vi "LVCAM Destroy Self.vi"(10 "Error":errorcluster, 11 "Self Actor in":refnum<class "Self Actor.lvclass">) -> (0 "error out":errorcluster, 1 "Destroyed Self?":bool, 3 "Self Actor out":refnum<class "Self Actor.lvclass">)   [LabVIEW 2021, in "LVCAM.lvlib" / "Self Actor.lvclass"]
uses:
  Self Actor.lvclass
  C:/PPLs/LabVIEW-Composed-Actor-Model-LVCAM/LabVIEW-Composed-Actor-Model-LVCAM/AAM/LVCAM/LVCAM/LVCAM.lvclass
  Self Actor.lvclass/Self Actor.ctl
  Msgs/LVCAM Destroy Self/LVCAM Destroy Self Msg/LVCAM Destroy Self Msg.lvclass
  C:/PPLs/LabVIEW-Composed-Actor-Model-LVCAM/LabVIEW-Composed-Actor-Model-LVCAM/AAM/LVCAM/Msg/Msg.lvclass
  Msgs/LVCAM Nest Destroyed/LVCAM Nest Destroyed Msg/LVCAM Nest Destroyed Msg.lvclass
  Nest Msg Send.vi
  Call Msg Send.vi
  Msg Q/Msg Q.lvclass
  C:/PPLs/LabVIEW-Composed-Actor-Model-LVCAM/LabVIEW-Composed-Actor-Model-LVCAM/AAM/Msgs/LVCAM Destroy Self/LVCAM Destroy Self Msg/LVCAM Destroy Self Msg.lvclass
  C:/PPLs/LabVIEW-Composed-Actor-Model-LVCAM/LabVIEW-Composed-Actor-Model-LVCAM/AAM/Msgs/LVCAM Destroy Self/LVCAM Destroy Self/LVCAM Destroy Self.lvclass
  C:/PPLs/LabVIEW-Composed-Actor-Model-LVCAM/LabVIEW-Composed-Actor-Model-LVCAM/AAM/Msgs/LVCAM Nest Destroyed/LVCAM Nest Destroyed Msg/LVCAM Nest Destroyed Msg.lvclass
  C:/PPLs/LabVIEW-Composed-Actor-Model-LVCAM/LabVIEW-Composed-Actor-Model-LVCAM/AAM/Msgs/LVCAM Nest Destroyed/LVCAM Nest Destroyed/LVCAM Nest Destroyed.lvclass
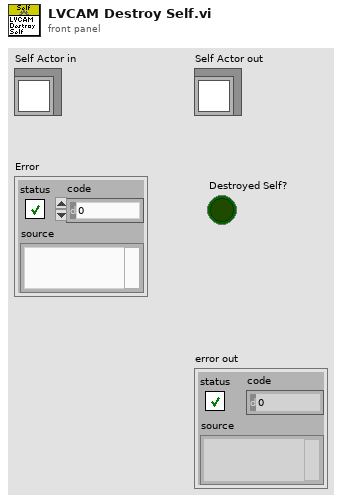
[diagram p1: front panel]
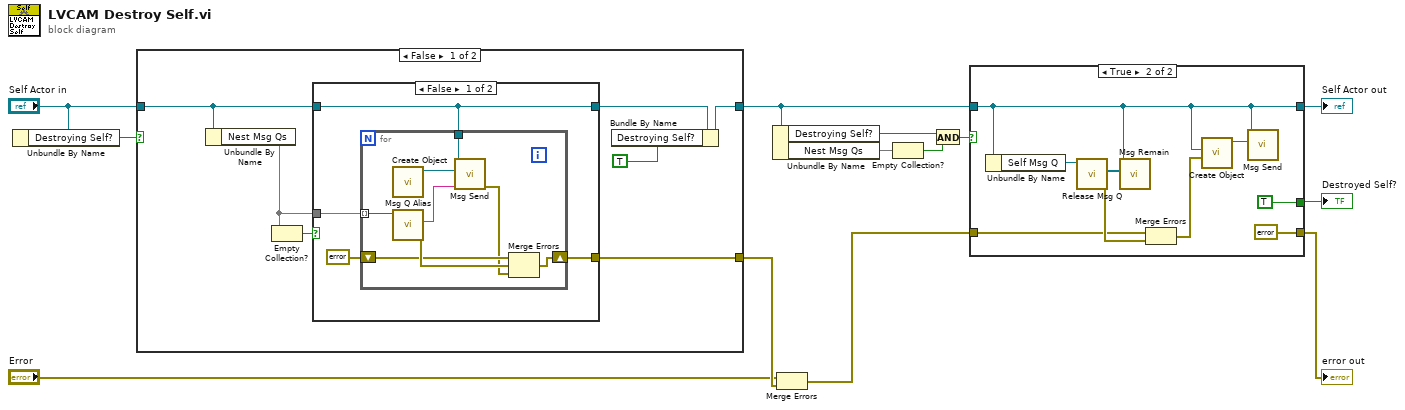
[diagram p0: block diagram]
diagram:
  n1 = Unbundle By Name("Self Actor in") -> ("Destroying Self?"=w10:bool)
  n2 = case shown="False" w10 {
    tunnel: [w18 _] -> w13
    tunnel: [w15 w34] -> w9
    tunnel: "Self Actor in" -> [w16 w34]
    frame False {
      n3 = Unbundle By Name(w16) -> ("Nest Msg Qs"=w19:set{refnum<class "Msg Q.lvclass">})
      n4 = Empty Collection?(1:w19) -> (0:w20:bool)
      n5 = case shown="False" w20 {
        tunnel: [w24 w33] -> w17
        tunnel: w16 -> [w24 w33]
        tunnel: w19 -> [w23 _]
        tunnel: [w22 _] -> w18
        frame False {
          n6 = for {
            tunnel: w24 -> [w28]
            tunnel: w23 -> [w32] mode=indexing
            shift-right: [w31] -> w22
            shift-left: errorcluster {"status"=FALSE, "code"=0, "source"=""} ("error out") -> [w29]
            n7 = call "Create Object.vi"() -> ("LVCAM Destroy Self Msg out"=w27:refnum<class "LVCAM Destroy Self Msg.lvclass">)  [unwired: 11 in]
            n8 = call "Msg Q Alias.vi"("Msg Q in"=w32) -> ("error out"=w30:errorcluster, "Msg Q Alias"=w26:string)  [unwired: 9 in]
            n9 = call-poly "Msg Send.vi"("Alias"=w26, "Msg"=w27, "Self Actor in"=w28) -> ("error out"=w25:errorcluster)  [unwired: 8 in]
            n10 = Merge Errors(w29, w30, w25) -> (w31:errorcluster)
          }
        }
        frame True {
        }
      }
      n11 = Bundle By Name(cluster=w17, "Destroying Self?"=TRUE) -> (w15:refnum<class "Self Actor.lvclass">)
    }
    frame True {
    }
  }
  n12 = Unbundle By Name(w9) -> ("Destroying Self?"=w4:bool, "Nest Msg Qs"=w8:set{refnum<class "Msg Q.lvclass">})
  n13 = Merge Errors("Error", w13) -> (w7:errorcluster)
  n14 = Empty Collection?(1:w8) -> (0:w5:bool)
  n15 = And(x=w4, y=w5) -> (x .and. y?=w6:bool)
  n16 = case shown="True" w6 {
    tunnel: w9 -> [w36 w40]
    tunnel: w7 -> [w35 w41]
    tunnel: [w36 w40] -> w3
    tunnel: [w35 errorcluster {"status"=FALSE, "code"=0, "source"=""} ("error IO")] -> w2
    tunnel: [_ TRUE ("Destroyed Self?")] -> w1
    frame False {
    }
    frame True {
      n17 = Unbundle By Name(w40) -> ("Self Msg Q"=w45:refnum<class "Msg Q.lvclass">)
      n18 = call "Release Msg Q.vi"("Msg Queue in"=w45) -> ("error out"=w42:errorcluster, "Remaining Elements"=w44:refnum<class "Msg.lvclass">[])  [unwired: 9 in]
      n19 = call-dynamic "Msg Remain.vi"("Remaining Elements"=w44, "Self Actor in"=w40) -> ()  [unwired: 10 in]
      n20 = Merge Errors(w41, w42) -> (w39:errorcluster)
      n21 = call "Create Object.vi"("Self Error"=w39, "Self Actor"=w40) -> ("LVCAM Nest Destroyed Msg out"=w43:refnum<class "LVCAM Nest Destroyed Msg.lvclass">)  [unwired: 9 in]
      n22 = call-poly "Msg Send.vi"("Msg"=w43, "Self Actor in"=w40) -> ()  [unwired: 9 in, 1 out]
    }
  }
  "error out" <- w2
  "Self Actor out" <- w3
  "Destroyed Self?" <- w1
